vi "attenuate.vi"(7 "auto":bool, 8 "Error in":errorcluster, 10 "Attenuate (dBm)":u32=10, 11 "VISA name in":refnum<visa-resource-name>) -> (0 "Error out":errorcluster, 3 "VISA name out":refnum<visa-resource-name>)   [LabVIEW 2012]
panel:
  out "cmd terminate":string
  out "cmd echo":string="\r\n"
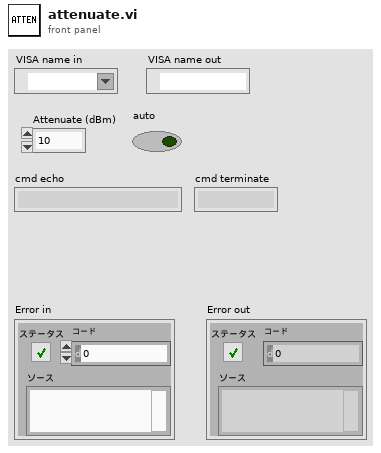
[diagram p1: front panel]
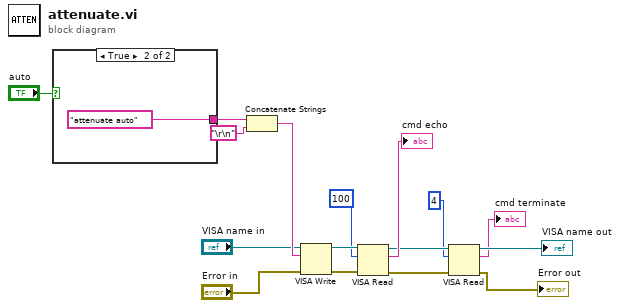
[diagram p0: block diagram]
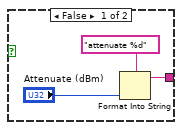
[diagram p2: hidden frame]
diagram:
  n1 = case shown="TRUE" "auto" {
    tunnel: [w19 "attenuate auto" ("形式文字列")] -> w7
    frame False {
      n2 = Format Into String(format string="attenuate %d" ("形式文字列"), "Attenuate (dBm)") -> (resulting string=w19:string)  [unwired: 2 in, 1 out]
    }
    frame True {
    }
  }
  n3 = Concatenate Strings(w7, "\r\n") -> (w15:string)
  n4 = VISA Write(VISA resource name="VISA name in", write buffer=w15, error in (no error)="Error in") -> (VISA resource name out=w13:refnum<visa-resource-name>, error out=w12:errorcluster)  [unwired: 1 out]
  n5 = VISA Read(VISA resource name=w13, byte count=u32 100 ("バイトカウント"), error in (no error)=w12) -> (VISA resource name out=w9:refnum<visa-resource-name>, read buffer=→"cmd echo":string, error out=w3:errorcluster)  [unwired: 1 out]
  n6 = VISA Read(VISA resource name=w9, byte count=u32 4 ("バイトカウント"), error in (no error)=w3) -> (VISA resource name out=→"VISA name out":refnum<visa-resource-name>, read buffer=→"cmd terminate":string, error out=→"Error out":errorcluster)  [unwired: 1 out]
